vi "总磷数据时间处理.vi"(9 "总磷修正数据输入":T1 {"单位" items=["ug/L", "mg/L", "ppm", "mg/m3", "cm", "ppb", "ug/m3", "%", "nmol/mol", "umol/mol", "MPN/L", "MPN/100ml", "ng/m3", "NTU", "无量纲", "ms/cm", "us/cm", "℃", "mV", "万个/L"]}, 10 "总磷原始数据":T1 {"单位" items=["ug/L", "mg/L", "ppm", "mg/m3", "cm", "ppb", "ug/m3", "%", "nmol/mol", "umol/mol", "MPN/L", "MPN/100ml", "ng/m3", "NTU", "无量纲", "ms/cm", "us/cm", "℃", "mV", "万个/L"]}, 11 "氨氮原始数据":T1 {"单位" items=["ug/L", "mg/L", "ppm", "mg/m3", "cm", "ppb", "ug/m3", "%", "nmol/mol", "umol/mol", "MPN/L", "MPN/100ml", "ng/m3", "NTU", "无量纲", "ms/cm", "us/cm", "℃", "mV", "万个/L"]}) -> (3 "氨氮修正数据输出":T1 {"单位" items=["ug/L", "mg/L", "ppm", "mg/m3", "cm", "ppb", "ug/m3", "%", "nmol/mol", "umol/mol", "MPN/L", "MPN/100ml", "ng/m3", "NTU", "无量纲", "ms/cm", "us/cm", "℃", "mV", "万个/L"]})   [LabVIEW 2016, in "氨氮总磷.lvlib"]
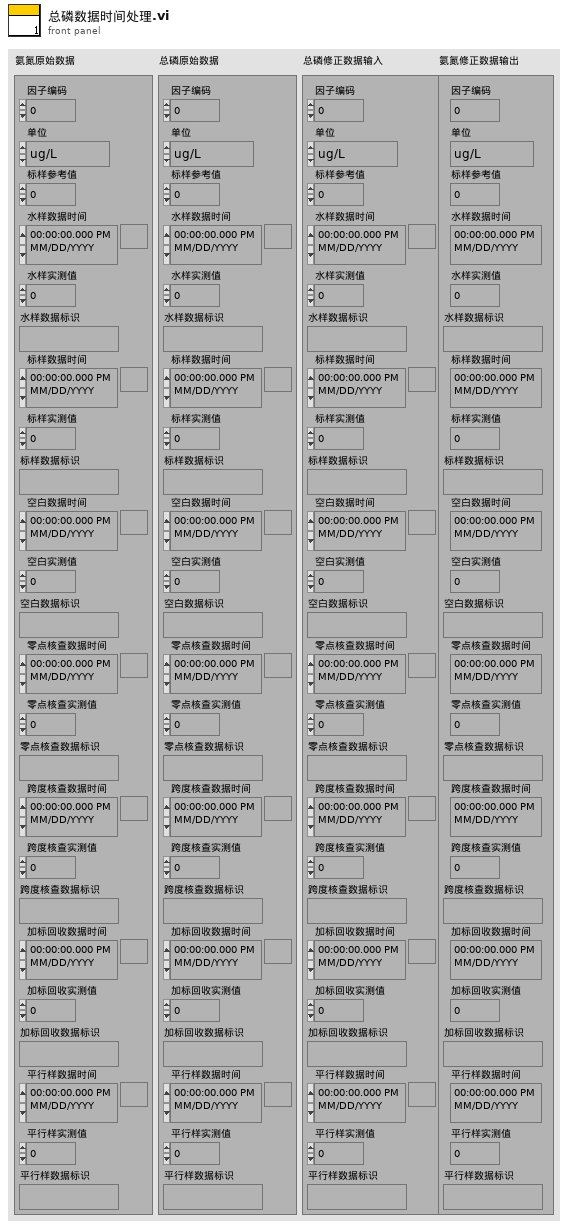
[diagram p1: front panel]
types:
  T1 = cluster{"因子编码":u32, "单位":u16, "标样参考值":sgl, "水样数据时间":timestamp, "水样实测值":sgl, "水样数据标识":string, "标样数据时间":timestamp, "标样实测值":sgl, "标样数据标识":string, "空白数据时间":timestamp, "空白实测值":sgl, "空白数据标识":string, "零点核查数据时间":timestamp, "零点核查实测值":sgl, "零点核查数据标识":string, "跨度核查数据时间":timestamp, "跨度核查实测值":sgl, "跨度核查数据标识":string, "加标回收数据时间":timestamp, "加标回收实测值":sgl, "加标回收数据标识":string, "平行样数据时间":timestamp, "平行样实测值":sgl, "平行样数据标识":string}
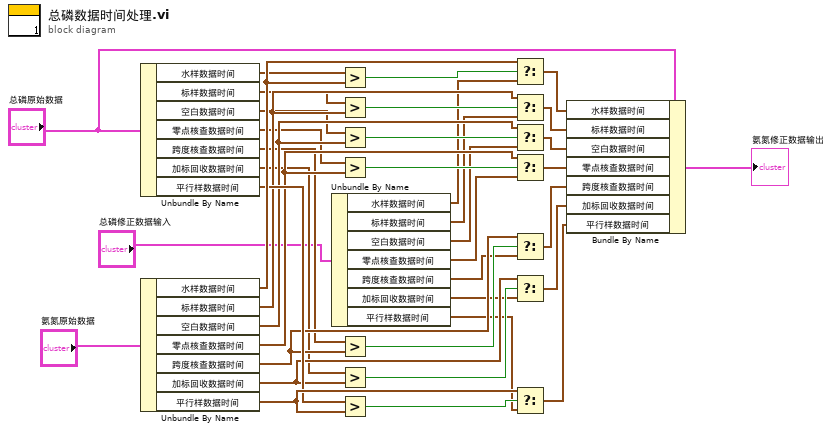
[diagram p0: block diagram]
diagram:
  n1 = Unbundle By Name("总磷原始数据") -> ("水样数据时间"=w37:timestamp, "标样数据时间"=w25:timestamp, "空白数据时间"=w22:timestamp, "零点核查数据时间"=w19:timestamp, "跨度核查数据时间"=w16:timestamp, "加标回收数据时间"=w12:timestamp, "平行样数据时间"=w33:timestamp)
  n2 = Unbundle By Name("氨氮原始数据") -> ("水样数据时间"=w38:timestamp, "标样数据时间"=w26:timestamp, "空白数据时间"=w23:timestamp, "零点核查数据时间"=w20:timestamp, "跨度核查数据时间"=w17:timestamp, "加标回收数据时间"=w13:timestamp, "平行样数据时间"=w34:timestamp)
  n3 = Unbundle By Name("总磷修正数据输入") -> ("水样数据时间"=w11:timestamp, "标样数据时间"=w10:timestamp, "空白数据时间"=w9:timestamp, "零点核查数据时间"=w8:timestamp, "跨度核查数据时间"=w7:timestamp, "加标回收数据时间"=w6:timestamp, "平行样数据时间"=w5:timestamp)
  n4 = Greater?(x=w37, y=w38) -> (0:w39:bool)
  n5 = Greater?(x=w25, y=w26) -> (0:w27:bool)
  n6 = Greater?(x=w22, y=w23) -> (0:w28:bool)
  n7 = Greater?(x=w19, y=w20) -> (0:w29:bool)
  n8 = Greater?(x=w16, y=w17) -> (0:w30:bool)
  n9 = Greater?(x=w12, y=w13) -> (0:w31:bool)
  n10 = Greater?(x=w33, y=w34) -> (0:w35:bool)
  n11 = Select(t=w38, s=w39, f=w11) -> (s? t:f=w36:timestamp)
  n12 = Select(t=w26, s=w27, f=w10) -> (s? t:f=w24:timestamp)
  n13 = Select(t=w23, s=w28, f=w9) -> (s? t:f=w21:timestamp)
  n14 = Select(t=w20, s=w29, f=w8) -> (s? t:f=w18:timestamp)
  n15 = Select(t=w17, s=w30, f=w7) -> (s? t:f=w15:timestamp)
  n16 = Select(t=w13, s=w31, f=w6) -> (s? t:f=w14:timestamp)
  n17 = Select(t=w34, s=w35, f=w5) -> (s? t:f=w32:timestamp)
  n18 = Bundle By Name(cluster="总磷原始数据", "水样数据时间"=w36, "标样数据时间"=w24, "空白数据时间"=w21, "零点核查数据时间"=w18, "跨度核查数据时间"=w15, "加标回收数据时间"=w14, "平行样数据时间"=w32) -> (→"氨氮修正数据输出":T1)
